vi "eHS Matrix Generation Main (Advanced).vi"(8 "Error In":errorcluster) -> (0 "error out":errorcluster)   [LabVIEW 2017]
doc: "Provides a template UI example which demonstrates how to incorporate the API in a more complex architecture (Queued Message Handler)."
uses:
  <vilib>/OPAL-RT/eHS Toolkit/eHS Matrix Generation/_Controls/eHS Core Index.ctl
  <vilib>/OPAL-RT/eHS Toolkit/eHS Matrix Generation/_Controls/eHS Form Factor.ctl
  <vilib>/OPAL-RT/eHS Toolkit/eHS Matrix Generation/_Controls/eHS Matrix Generation Session.ctl
  <vilib>/OPAL-RT/eHS Toolkit/eHS Matrix Generation/_Controls/eHS Target Information.ctl
  <vilib>/OPAL-RT/eHS Toolkit/eHS Matrix Generation/_Controls/eHS Matrix Generation Parameters.ctl
  <vilib>/OPAL-RT/eHS Toolkit/eHS Matrix Generation/_Controls/eHS Circuit Analysis Data.ctl
  <vilib>/OPAL-RT/eHS Toolkit/eHS Matrix Generation/_Controls/eHS Core Settings.ctl
  <vilib>/OPAL-RT/eHS Toolkit/eHS Matrix Generation/_Controls/eHS Model Information.ctl
  Controls/UI Data.ctl
  Controls/General UI Refs.ctl
  Controls/Info Extraction UI Refs.ctl
  Controls/Session Init UI Refs.ctl
  Controls/Matrix Gen UI Refs.ctl
  Controls/Session Reset_Close UI Refs.ctl
  Controls/Info to Add Model.ctl
  Support/ListBox/ListBox Action.ctl
  Support/Message Queue/Enqueue Message (Single).vi
  <vilib>/Utility/error.llb/Error Cluster From Error Code.vi
  <vilib>/ErrorRing/Error Ring.xnode
  Support/Message Queue/Message Queue.lvlib
  Support/User Event - Stop/User Event - Stop.lvlib
  <vilib>/OPAL-RT/eHS Toolkit/eHS Matrix Generation/eHS Matrix Generation.lvlib
panel:
  in  "TAB":T1(tab) caption="DC Source"
  in  "Add Model(s)-File":bool
  in  "eHS Listbox":i32(listbox)
  in  "Close Session":bool
  in  "Extract Model(s) Info":bool
  in  "Generate Matrix(s)":bool
  in  "Support Scenarios?":bool
  in  "Transfer Matrices":bool
  in  "Update Settings":bool
  in  "eHS Form Factor":T2=enum."eHSx64"
  in  "eHS Core Index":T3
  in  "Model Location On Disk":path
  in  "Add Model":bool
  in  "Create Session":bool
  in  "Reset Session":bool
  in  "Quit Button":bool
  in  "Target Password":string
  in  "Target Username":string="admin"
  in  "Help Button":bool
  out "?":string
  in  "Deployment Target":refnum<k21>
  in  "Get Report":bool
  out "eHS Generation Reports":string
  # "Deployment Target Settings"
  # "Model Information"
  # "Step 1: Create a session by selecting a deployment target (username and password if applicable) and click on Create Session.\nStep 2: Select *.mdl, *.slx, *.psimsch, *.cct or NI Multisim *.xml file. In addition, choose the eHS Form Factor for the generation and a Core Index for this model. \nYou can use this core index throughout the application to refer to a specific model.\nStep 3: Click on Add Model to add this model to the eHS Matrix Generation session.\nStep 4: Repeat step 2 & 3 if you want to generate more then one eHS matrix.\nStep 5: Click on Extract Model(s). This can take several minutes. The information extraction results will be displayed in the consoles to the right.\nStep 6 (Optional): Press the Update Settings button to change some of the matrix generation parameters before generating them.\nStep 7: Click on Generate Matrix(s). A eHS matrix will be generated for each model that was loaded into the session.\nStep 8: Once the matrices have been generated, you can transfer the matrices to the deplayment target by clicking on the Transfer Matrices button. \nStep 9: At this point, you can update the setting and generate a new set of matrices (Update Settings), you can reset the session (Reset Session), you can close \nthe current session (Close Session), or you can stop the application (Quit). \n \nBefore running this VI please note that:\n\n1- Before starting the real-time simulation, users need to define the circuit configuration, using an appropriate circuit editor. \nThe following circuit editors are supported by OPAL-RT TECHNOLOGIES:           \n                - Matlab/Simulink SimPowwerSystems (SPS)  (*.mdl or *.slx)\n                - Matlab/Simulink PLECS blockset  (*.mdl or *.slx)\n                - PSIM  (*.psimsch or *.cct)\n                - NI Multisim (xml output *.xml)\n\n2- PSIM and NI Multisim users have to install\t32-bit version of MATLAB® Runtime version 9.0 (R2015b) availible at:\n                                 http://www.mathworks.com/products/compiler/mcr/index.html\n\n3- Please also note that you need to have valid licence of one of the mentioned circuit editors to be able to generate the eSH matrix. In other words the users \nwho want to select SimPowerSystem (SPS) model must be have valid licence of Matlab/Simulink and SPS toolbox, the users who want to select PLECS blockset \nmodel must be have valid licence of Matlab/Simulink and PLECS blockset, the users who want to select PSIM model must be have valid licence off PSIM, and the users who want to generate and select the NI Multism xml file must be have valid licence of NI Multisim. If you don't have valid license of the \nmentioned circuit editors, you can only select prebuilt xml files."
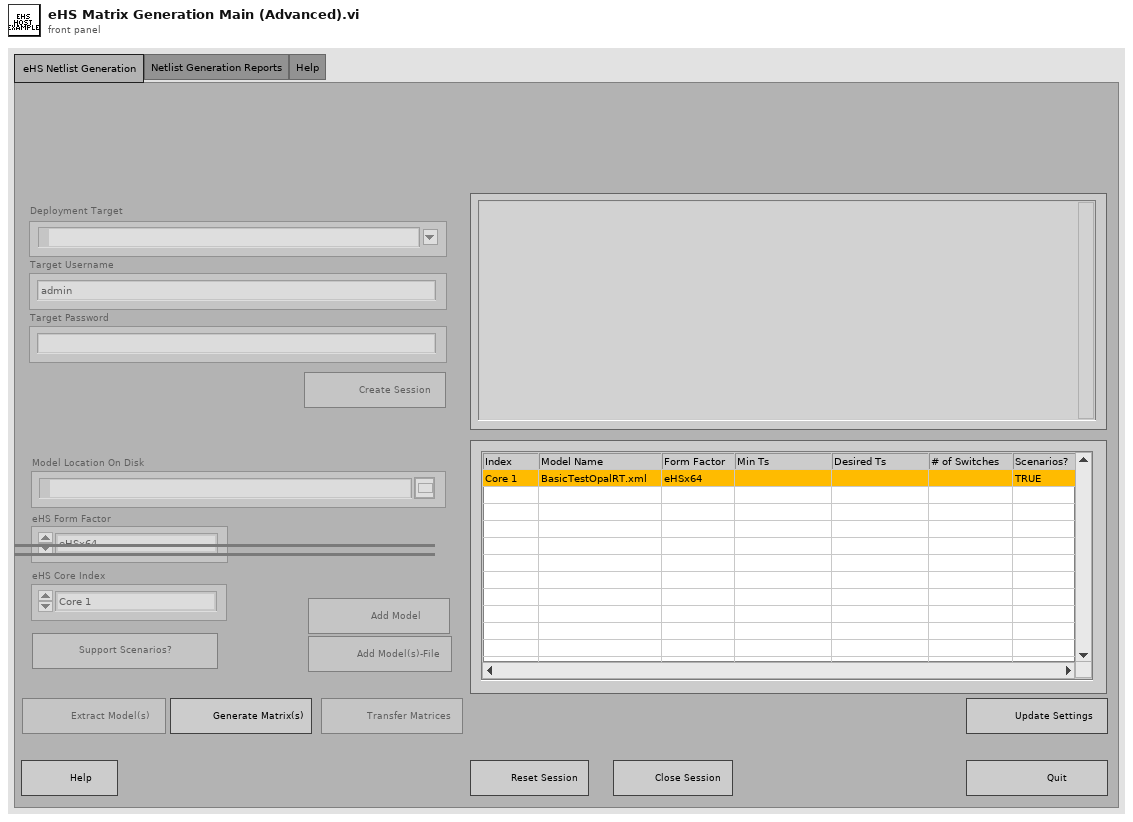
[diagram p1: front panel]
types:
  T1 = enum32{"eHS Netlist Generation ", "Netlist Generation Reports", "Help"}
  T2 = typedef "OPAL-RT eHS.lvlib/eHS Matrix Generation.lvlib/eHS Form Factor.ctl" = enum16{"eHSx16", "eHSx32", "eHSx64"}
  T3 = typedef "OPAL-RT eHS.lvlib/eHS Matrix Generation.lvlib/eHS Core Index.ctl" = enum16{"Core 1", "Core 2", "Core 3", "Core 4", "Core 5", "Core 6", "Core 7", "Core 8", "Core 9", "Core 10"}
  T4 = typedef "UI Data.ctl" = cluster{"Transfer Netlist(s)":refnum<vi>, "General Refs":T5, "Info Extraction Refs":T6, "Session Init Refs":T7, "Matrix Gen Refs":T8, "Session R\\C Refs":T9, "eHS Listbox":refnum<vi>}
  T5 = typedef "General UI Refs.ctl" = cluster{"Help":refnum<vi>, "Quit":refnum<vi>}
  T6 = typedef "Info Extraction UI Refs.ctl" = cluster{"Support Scenarios?":refnum<vi>, "Add Model":refnum<vi>, "Extract Model(s) Info":refnum<vi>, "Model Location":refnum<vi>, "Add Model(s)-File":refnum<vi>, "eHS Core Index":refnum<vi>, "eHS Form Factor":refnum<vi>}
  T7 = typedef "Session Init UI Refs.ctl" = cluster{"Create Session":refnum<vi>, "Password":refnum<vi>, "Username":refnum<vi>, "Deployment Target":refnum<vi>}
  T8 = typedef "Matrix Gen UI Refs.ctl" = cluster{"Update Settings":refnum<vi>, "Generate Matrix(s)":refnum<vi>}
  T9 = typedef "Session Reset_Close UI Refs.ctl" = cluster{"Reset Session":refnum<vi>, "Close Session":refnum<vi>}
  T10 = typedef "OPAL-RT eHS.lvlib/eHS Matrix Generation.lvlib/eHS Target Information.ctl" = cluster{"Deployment Target":refnum<k21>, "Username":string, "Password":string}
  T11 = typedef "Info to Add Model.ctl" = cluster{"eHS Core Settings":T12, "eHS Model Information":T13}
  T12 = typedef "OPAL-RT eHS.lvlib/eHS Matrix Generation.lvlib/eHS Core Settings.ctl" = cluster{"eHS Form Factor":T2, "eHS Core Index":T3}
  T13 = typedef "OPAL-RT eHS.lvlib/eHS Matrix Generation.lvlib/eHS Model Information.ctl" = cluster{"Model File Path":path, "Model Name":string, "Model File Extension":string, "Senarios?":bool}
  T14 = enum8{"Enabled", "Disabled", "Disabled and Grayed Out"}
  T15 = typedef "ListBox Action.ctl" = enum16{"Add", "Overwrite"}
  T16 = typedef "Message Queue.lvlib/All Message Queues.ctl" = cluster{"UI":refnum<queue>}
  T17 = typedef "OPAL-RT eHS.lvlib/eHS Matrix Generation.lvlib/eHS Circuit Analysis Data.ctl" = cluster{"Number of Switches":string, "Desired Ts":string, "Gs":dbl[], "Min Ts":string}
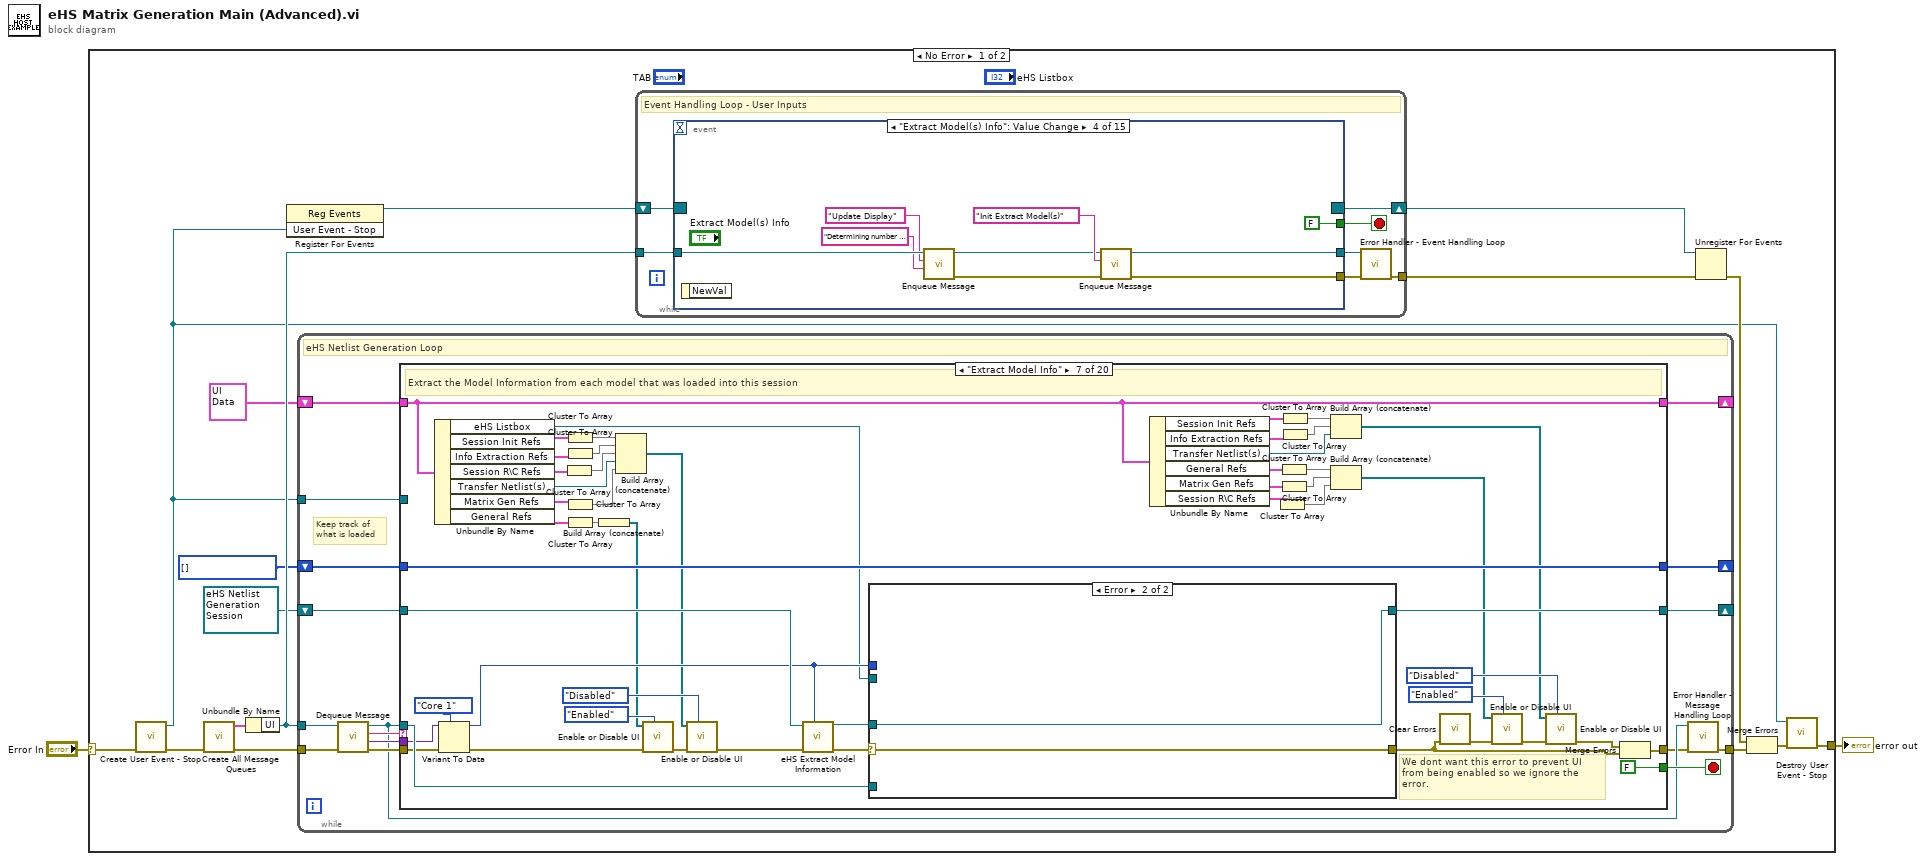
[diagram p0: block diagram]
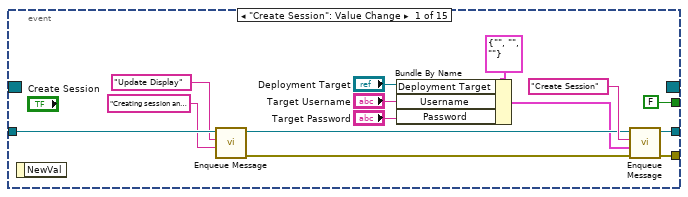
[diagram p2: hidden frame]
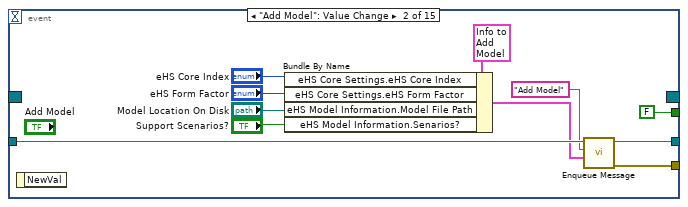
[diagram p3: hidden frame]
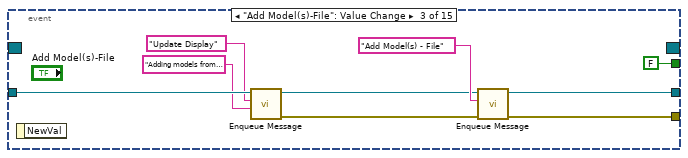
[diagram p4: hidden frame]
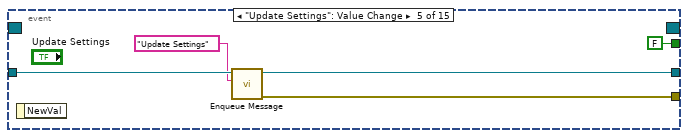
[diagram p5: hidden frame]
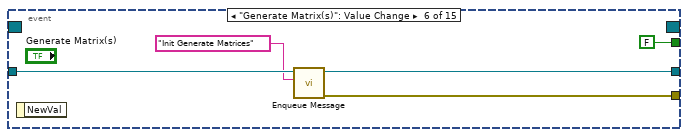
[diagram p6: hidden frame]
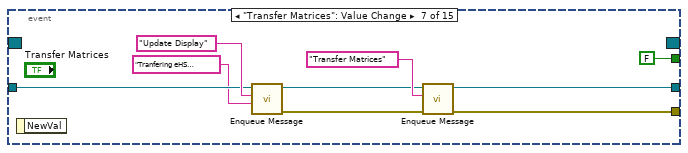
[diagram p7: hidden frame]
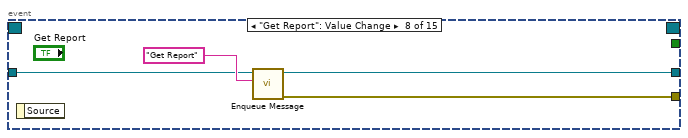
[diagram p8: hidden frame]
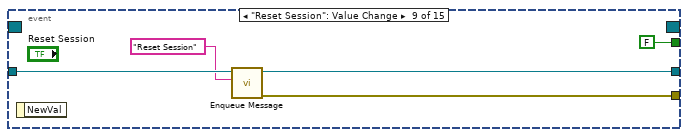
[diagram p9: hidden frame]
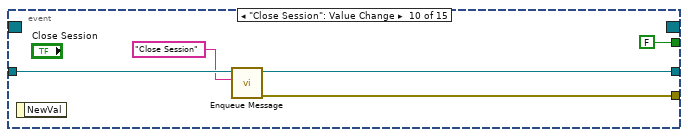
[diagram p10: hidden frame]
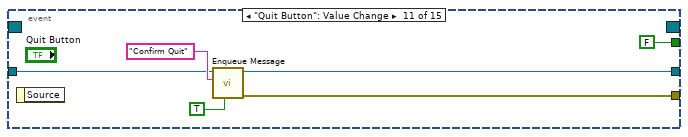
[diagram p11: hidden frame]
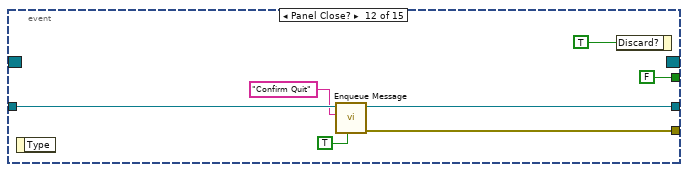
[diagram p12: hidden frame]
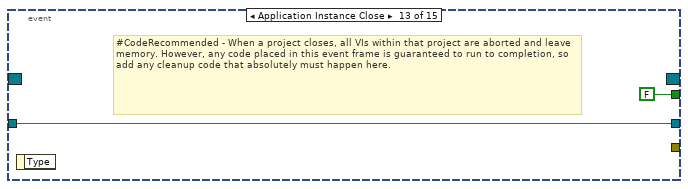
[diagram p13: hidden frame]
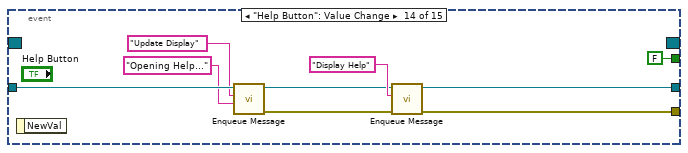
[diagram p14: hidden frame]
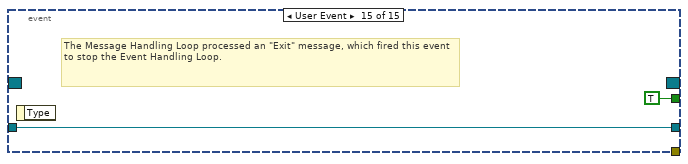
[diagram p15: hidden frame]
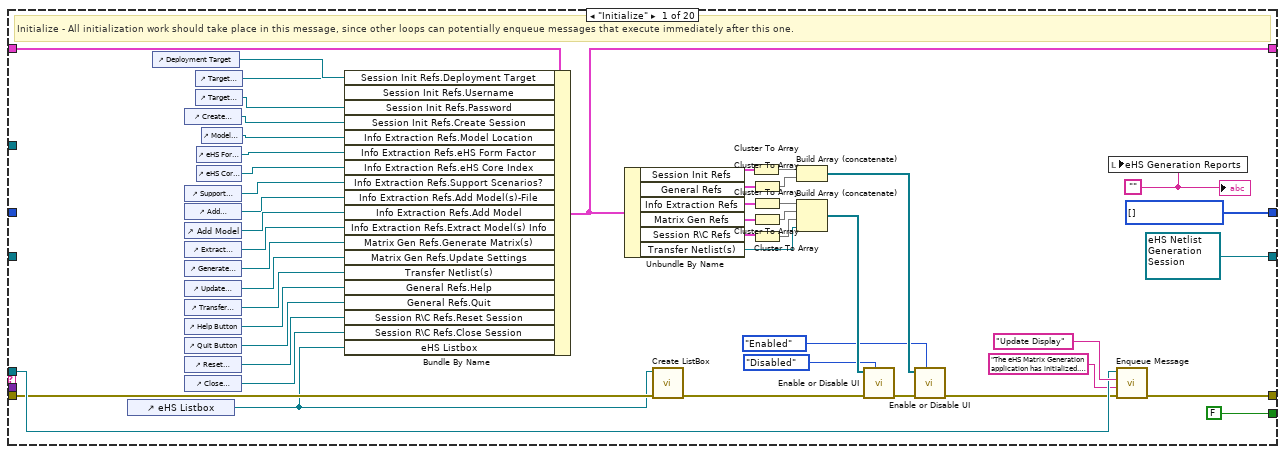
[diagram p16: hidden frame]
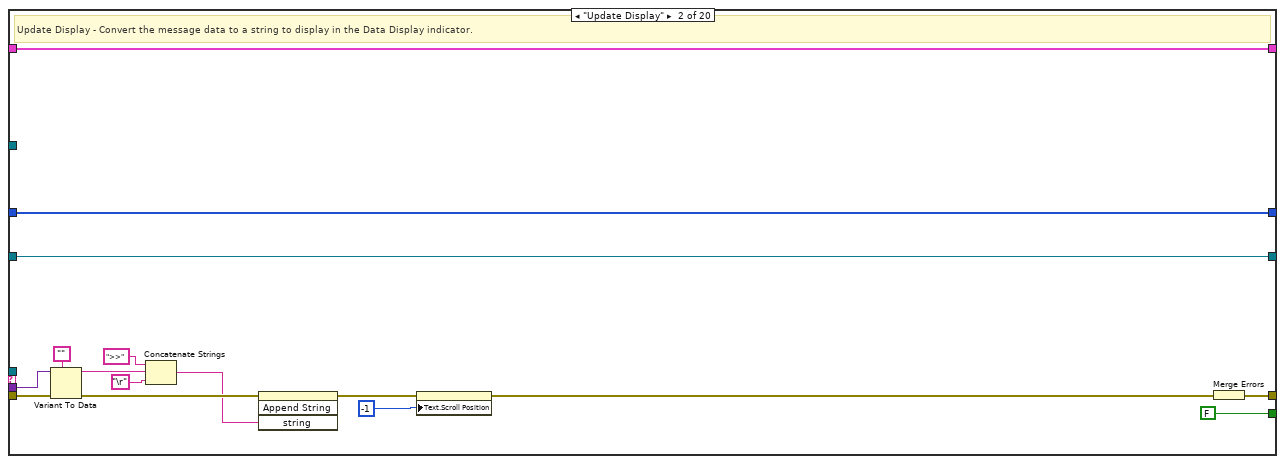
[diagram p17: hidden frame]
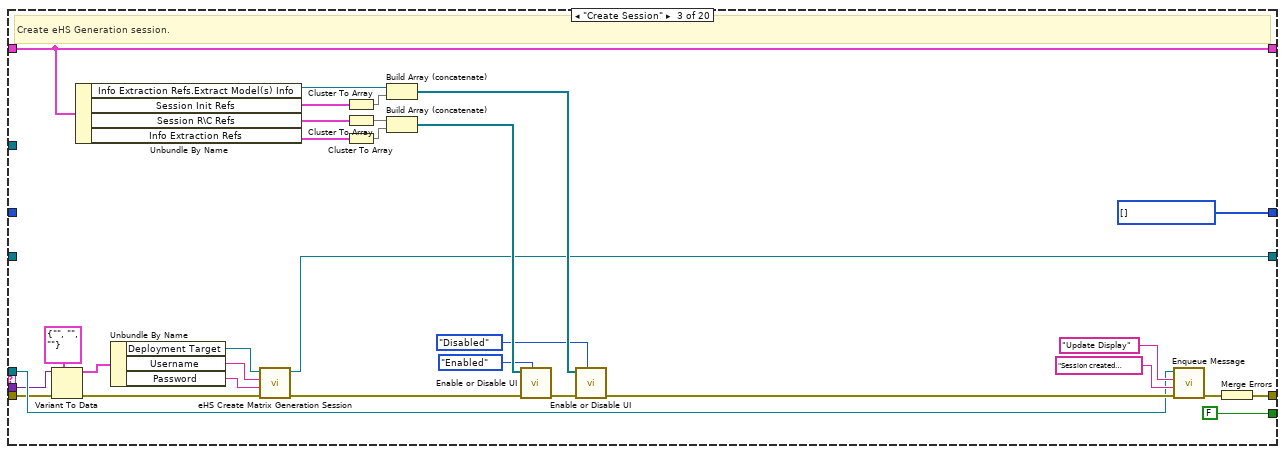
[diagram p18: hidden frame]
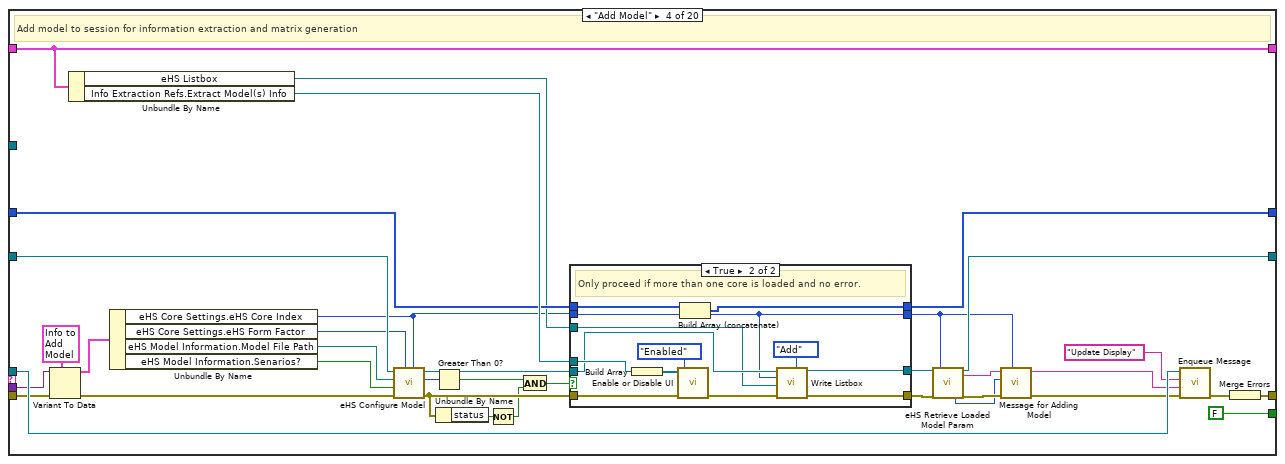
[diagram p19: hidden frame]
diagram:
  n1 = case shown="No Error" "Error In" {
    selector: "Error In" -> [w3 w781]
    tunnel: [w4 w781] -> w2
    frame No Error {
      w5 = T3[] [] items=["Core 1", "Core 2", "Core 3", "Core 4", "Core 5", "Core 6", "Core 7", "Core 8", "Core 9", "Core 10"]
      n2 = call "Create User Event - Stop.vi"("Error In"=w3) -> ("Error out"=w14:errorcluster, "User Event - Stop"=w8:refnum<user-event>)  [unwired: 9 in]
      n3 = call "Create All Message Queues.vi"("Error In"=w14) -> ("Error Out"=w18:errorcluster, "Message Queues Out"=w17:T16)  [unwired: 9 in]
      n4 = Unbundle By Name(w17) -> ("UI"=w15:refnum<queue>)
      n5 = register-events(w8) -> (reference out=w9:refnum<event-registration>)  [unwired: 2 in, 1 out]
      n6 = while {
        tunnel: w15 -> [w135]
        shift-right: [w142] -> _
        shift-left: T4 {"Transfer Netlist(s)"=refnum, "General Refs"={"Help"=refnum, "Quit"=refnum}, "Info Extraction Refs"={"Support Scenarios?"=refnum, "Add Model"=refnum, "Extract Model(s) Info"=refnum, "Model Location"=refnum, "Add Model(s)-File"=refnum, "eHS Core Index"=refnum, "eHS Form Factor"=refnum}, "Session Init Refs"={"Create Session"=refnum, "Password"=refnum, "Username"=refnum, "Deployment Target"=refnum}, "Matrix Gen Refs"={"Update Settings"=refnum, "Generate Matrix(s)"=refnum}, "Session R\\C Refs"={"Reset Session"=refnum, "Close Session"=refnum}, "eHS Listbox"=refnum} ("Data Cluster") -> [w143]
        tunnel: w8 -> [w140]
        tunnel: w18 -> [w139]
        tunnel: [w133] -> w16
        shift-right: [w130] -> _
        shift-left: refnum<data-value> refnum ("eHS Matrix Generation Session Ref") -> [w131]
        shift-right: [w128] -> _
        shift-left: w5 -> [w129]
        stop <- w141 stop-if-true
        # "Keep track of \nwhat is loaded"
        # "eHS Netlist Generation Loop"
        n7 = call "Dequeue Message.vi"("error in (no error)"=w139, "Message Queue"=w135) -> ("error out"=w138:errorcluster, "Message Data"=w136:variant, "Message"=w137:string, "dup Message Queue"=w134:refnum<queue>)  [unwired: 6 in]
        n8 = case "Message Cases" shown="\"Extract Model Info\"" w137 {
          selector: w137 -> [_ _ _ _ _ _ _ _ _ _ _ _ _ _ _ _ _ _ _ w771]
          tunnel: w134 -> [w188 _ w222 w270 w307 w342 w413 w450 w500 w547 w585 w645 w679 w699 _ w732 w753 _ _ _]
          tunnel: w138 -> [w148 w205 w215 w247 w312 w349 w412 w475 w507 w567 w617 w640 w675 w702 w719 w731 w748 w763 w767 _]
          tunnel: [w191 w206 w238 w274 w315 w363 w371 w445 w520 w575 w586 w661 w695 w700 w723 w739 w751 w757 w765 w772] -> w132
          tunnel: w143 -> [w190 w207 w228 w265 w302 w352 w389 w461 w510 w538 w595 w642 w677 w706 w724 w740 w752 w762 w766 w773]
          tunnel: [w171 w207 w228 w265 w302 w352 w389 w461 w510 w538 w595 w642 w677 w706 w724 w740 w752 w762 w766 w773] -> w142
          tunnel: [FALSE FALSE FALSE FALSE FALSE FALSE FALSE FALSE FALSE FALSE FALSE FALSE FALSE _ FALSE FALSE TRUE FALSE FALSE FALSE] -> w141
          tunnel: w136 -> [_ w204 w212 w245 _ _ w411 _ _ w566 _ _ _ _ _ _ w745 w761 _ _]
          tunnel: w140 -> [_ _ _ _ _ _ _ _ _ _ _ _ _ _ _ _ w750 _ _ _]
          tunnel: w131 -> [_ w199 _ w272 w313 w345 w416 w485 w503 w569 w612 w641 w676 w697 w720 w735 _ w755 _ w768]
          tunnel: [refnum<data-value> refnum ("eHS Matrix Generation Session Ref") w199 w220 w259 w303 w345 w415 w484 w503 w568 w611 w638 refnum<data-value> refnum ("eHS Matrix Generation Session Ref") w697 w720 w735 refnum<data-value> refnum ("eHS Matrix Generation Session Ref") w755 _ w768] -> w130
          tunnel: w129 -> [_ w198 _ w262 _ w343 w408 w453 w501 w570 w610 _ _ w696 w721 w725 _ w754 _ w769]
          tunnel: [w149 w198 w216 w263 w295 w343 w408 w453 w501 w570 w610 w636 w666 w696 w721 w725 w741 w754 _ w769] -> w128
          frame "Initialize" {
            w149 = T3[] [] items=["Core 1", "Core 2", "Core 3", "Core 4", "Core 5", "Core 6", "Core 7", "Core 8", "Core 9", "Core 10"]
            w144 = ""
            # "Initialize - All initialization work should take place in this message, since other loops can potentially enqueue messages that execute immediately after this one."
            n9 = control-ref of="eHS Listbox"() -> (w146:refnum<vi>)
            n10 = control-ref of="Deployment Target"() -> (w186:refnum<vi>)
            n11 = control-ref of="Create Session"() -> (w183:refnum<vi>)
            n12 = control-ref of="Support Scenarios?"() -> (w179:refnum<vi>)
            n13 = control-ref of="Add Model(s)-File"() -> (w145:refnum<vi>)
            n14 = control-ref of="Add Model"() -> (w178:refnum<vi>)
            n15 = control-ref of="Extract Model(s) Info"() -> (w177:refnum<vi>)
            n16 = control-ref of="Generate Matrix(s)"() -> (w176:refnum<vi>)
            n17 = control-ref of="Update Settings"() -> (w175:refnum<vi>)
            n18 = control-ref of="Transfer Matrices"() -> (w174:refnum<vi>)
            n19 = control-ref of="Help Button"() -> (w173:refnum<vi>)
            n20 = control-ref of="Quit Button"() -> (w172:refnum<vi>)
            n21 = control-ref of="Reset Session"() -> (w156:refnum<vi>)
            n22 = control-ref of="Close Session"() -> (w155:refnum<vi>)
            n23 = control-ref of="Target Username"() -> (w185:refnum<vi>)
            n24 = control-ref of="Target Password"() -> (w184:refnum<vi>)
            n25 = control-ref of="eHS Form Factor"() -> (w181:refnum<vi>)
            n26 = control-ref of="eHS Core Index"() -> (w180:refnum<vi>)
            n27 = control-ref of="Model Location On Disk"() -> (w182:refnum<vi>)
            n28 = Bundle By Name(cluster=w190, "Session Init Refs.Deployment Target"=w186, "Session Init Refs.Username"=w185, "Session Init Refs.Password"=w184, "Session Init Refs.Create Session"=w183, "Info Extraction Refs.Model Location"=w182, "Info Extraction Refs.eHS Form Factor"=w181, "Info Extraction Refs.eHS Core Index"=w180, "Info Extraction Refs.Support Scenarios?"=w179, "Info Extraction Refs.Add Model(s)-File"=w145, "Info Extraction Refs.Add Model"=w178, "Info Extraction Refs.Extract Model(s) Info"=w177, "Matrix Gen Refs.Generate Matrix(s)"=w176, "Matrix Gen Refs.Update Settings"=w175, "Transfer Netlist(s)"=w174, "General Refs.Help"=w173, "General Refs.Quit"=w172, "Session R\\C Refs.Reset Session"=w156, "Session R\\C Refs.Close Session"=w155, "eHS Listbox"=w146) -> (w171:T4)
            n29 = Unbundle By Name(w171) -> ("Session Init Refs"=w169:T7, "General Refs"=w170:T5, "Info Extraction Refs"=w168:T6, "Matrix Gen Refs"=w153:T8, "Session R\\C Refs"=w152:T9, "Transfer Netlist(s)"=w154:refnum<vi>)
            n30 = call "Create ListBox.vi"("Error In"=w148, "Multicolumn Listbox Ref In"=w146) -> ("Error Out"=w147:errorcluster)  [unwired: 8 in, 1 out]
            n31 = Cluster To Array(cluster=w169) -> (array=w167:refnum<vi>[])
            n32 = Cluster To Array(cluster=w170) -> (array=w166:refnum<vi>[])
            n33 = Cluster To Array(cluster=w168) -> (array=w164:refnum<vi>[])
            n34 = Cluster To Array(cluster=w153) -> (array=w165:refnum<vi>[])
            n35 = Cluster To Array(cluster=w152) -> (array=w151:refnum<vi>[])
            n36 = Build Array (concatenate)(w167, w166) -> (w159:refnum<vi>[])
            n37 = Build Array (concatenate)(w164, w165, w151, w154) -> (w163:refnum<vi>[])
            n38 = call "Enable or Disable UI.vi"("Action"=T14."Disabled", "Error In"=w147, "Control Refs"=w163) -> ("Error Out"=w161:errorcluster)  [unwired: 8 in]
            n39 = call "Enable or Disable UI.vi"("Action"=T14."Enabled", "Error In"=w161, "Control Refs"=w159) -> ("Error Out"=w160:errorcluster)  [unwired: 8 in]
            n40 = local write "eHS Generation Reports"(w144) -> ()
            n41 = call-poly "Enqueue Message.vi"("Error In"=w160, "Message Data"="The eHS Matrix Generation application has initialized. Please create a new session." ("Initial Message"), "Message"="Update Display", "Message Queue"=w188) -> ("Error Out"=w191:errorcluster)  [unwired: 6 in, 1 out]
            "?" <- w144
          }
          frame "Update Display" {
            # "Update Display - Convert the message data to a string to display in the Data Display indicator."
            n42 = Variant To Data(error in=w205, type="", Variant=w204) -> (data=w202:string, error out=w196:errorcluster)
            n43 = Concatenate Strings(">>" ("string"), w202, "\r") -> (w195:string)
            n44 = invoke class="Str" method="Append String"(error in=w196, "string"=w195) -> (error out=w194:errorcluster)  [unwired: 2 in, 3 out]
            n45 = property class="Str"(error in=w194, "Text.Scroll Position"=-1) -> (error out=w193:errorcluster)  [unwired: 1 in, 1 out]
            n46 = Merge Errors(w193) -> (w206:errorcluster)
          }
          frame "Create Session" {
            w216 = T3[] [] items=["Core 1", "Core 2", "Core 3", "Core 4", "Core 5", "Core 6", "Core 7", "Core 8", "Core 9", "Core 10"]
            # "Create eHS Generation session."
            n47 = Variant To Data(error in=w215, type=T10 {"Deployment Target"="", "Username"="", "Password"=""} ("eHS Target Information"), Variant=w212) -> (data=w211:T10, error out=w214:errorcluster)
            n48 = Unbundle By Name(w228) -> ("Info Extraction Refs.Extract Model(s) Info"=w217:refnum<vi>, "Session Init Refs"=w234:T7, "Session R\\C Refs"=w226:T9, "Info Extraction Refs"=w219:T6)
            n49 = Unbundle By Name(w211) -> ("Deployment Target"=w210:refnum<k21>, "Username"=w209:string, "Password"=w208:string)
            n50 = call <vilib>:"eHS Create Matrix Generation Session.vi"("Error In"=w214, "Target Password"=w208, "Target Username"=w209, "Deployment Target"=w210) -> ("Error Out"=w221:errorcluster, "eHS Matrix Generation Session Ref"=w220:refnum<data-value>)  [unwired: 6 in]
            n51 = Cluster To Array(cluster=w234) -> (array=w233:refnum<vi>[])
            n52 = Cluster To Array(cluster=w226) -> (array=w225:refnum<vi>[])
            n53 = Cluster To Array(cluster=w219) -> (array=w218:refnum<vi>[])
            n54 = Build Array (concatenate)(w217, w233) -> (w230:refnum<vi>[])
            n55 = Build Array (concatenate)(w225, w218) -> (w232:refnum<vi>[])
            n56 = call "Enable or Disable UI.vi"("Action"=T14."Enabled", "Error In"=w221, "Control Refs"=w232) -> ("Error Out"=w227:errorcluster)  [unwired: 8 in]
            n57 = call "Enable or Disable UI.vi"("Action"=T14."Disabled", "Error In"=w227, "Control Refs"=w230) -> ("Error Out"=w223:errorcluster)  [unwired: 8 in]
            n58 = call-poly "Enqueue Message.vi"("Error In"=w223, "Message Data"="Session created successfully. Ready to add models for matrix generation." ("Message"), "Message"="Update Display", "Message Queue"=w222) -> ("Error Out"=w224:errorcluster)  [unwired: 6 in, 1 out]
            n59 = Merge Errors(w224) -> (w238:errorcluster)
          }
          frame "Add Model" {
            # "Add model to session for information extraction and matrix generation"
            n60 = Variant To Data(error in=w247, type=T11 {"eHS Core Settings"={"eHS Form Factor"=enum."eHSx16", "eHS Core Index"=enum."Core 1"}, "eHS Model Information"={"Model File Path"=path "", "Model Name"="", "Model File Extension"="", "Senarios?"=FALSE}} ("Info to Add Model"), Variant=w245) -> (data=w243:T11, error out=w246:errorcluster)
            n61 = Unbundle By Name(w265) -> ("eHS Listbox"=w248:refnum<vi>, "Info Extraction Refs.Extract Model(s) Info"=w264:refnum<vi>)
            n62 = Unbundle By Name(w243) -> ("eHS Core Settings.eHS Core Index"=w242:T3, "eHS Core Settings.eHS Form Factor"=w241:T2, "eHS Model Information.Model File Path"=w240:path, "eHS Model Information.Senarios?"=w239:bool)
            n63 = call <vilib>:"eHS Configure Model.vi"("eHS Core Index"=w242, "eHS Form Factor"=w241, "Error In"=w246, "Support Senarios?"=w239, "Model File Path"=w240, "eHS Matrix Generation Session Ref In"=w272) -> ("Error Out"=w253:errorcluster, "Number of Cores Loaded"=w266:i32, "eHS Matrix Generation Session Ref Out"=w249:refnum<data-value>)  [unwired: 3 in]
            n64 = Greater Than 0?(x=w266) -> (x > 0?=w255:bool)
            n65 = Unbundle By Name(w253) -> ("status"=w252:bool)
            n66 = Not(x=w252) -> (.not. x?=w251:bool)
            n67 = And(x=w255, y=w251) -> (x .and. y?=w254:bool)
            n68 = case shown="True" w254 {
              tunnel: w242 -> [w276 w281]
              tunnel: w262 -> [w278 w291]
              tunnel: [w278 w290] -> w263
              tunnel: w253 -> [w277 w288]
              tunnel: [w277 w284] -> w261
              tunnel: w264 -> [_ w286]
              tunnel: [w276 w281] -> w256
              tunnel: [w275 w283] -> w250
              tunnel: w249 -> [w275 w282]
              tunnel: w248 -> [_ w280]
              frame False {
                # "Do nothing if no cores are loaded or error"
              }
              frame True {
                # "Only proceed if more than one core is loaded and no error."
                n69 = Build Array(w286) -> (w289:refnum<vi>[])
                n70 = call "Enable or Disable UI.vi"("Action"=T14."Enabled", "Error In"=w288, "Control Refs"=w289) -> ("Error Out"=w285:errorcluster)  [unwired: 8 in]
                n71 = Build Array (concatenate)(w291, w281) -> (w290:T3[])
                n72 = call "Write Listbox.vi"("Action"=ListBox_Action."Add" ("ListBox Action"), "eHS Core Index"=w281, "Error In"=w285, "Multicolumn Listbox Ref In"=w280, "eHS Matrix Generation Session Ref In"=w282) -> ("Error Out"=w284:errorcluster, "eHS Matrix Generation Session Ref Out"=w283:refnum<data-value>)  [unwired: 4 in, 1 out]
              }
            }
            n73 = call <vilib>:"eHS Retrieve Loaded Model Param.vi"("eHS Matrix Generation Session Ref In"=w250, "Error In"=w261, "eHS Core Index"=w256) -> ("Number of Loaded Models"=w257:i32, "eHS Matrix Generation Session Ref Out"=w259:refnum<data-value>, "Model Name"=w258:string, "Error Out"=w260:errorcluster)  [unwired: 10 in, 3 out]
            n74 = call "Message for Adding Model.vi"("eHS Core Index"=w256, "Error In"=w260, "Number of Loaded Models"=w257, "Model File Name"=w258) -> ("Error Out"=w267:errorcluster, "Message"=w268:string)  [unwired: 6 in]
            n75 = call-poly "Enqueue Message.vi"("Error In"=w267, "Message Data"=w268, "Message"="Update Display", "Message Queue"=w270) -> ("Error Out"=w271:errorcluster)  [unwired: 6 in, 1 out]
            n76 = Merge Errors(w271) -> (w274:errorcluster)
          }
          frame "Add Model(s) - File" {
            # "Duplicate this frame when creating new messages.  Change this comment in the duplicated frame to describe this message."
            n77 = Unbundle By Name(w302) -> ("Info Extraction Refs.Extract Model(s) Info"=w301:refnum<vi>, "eHS Listbox"=w293:refnum<vi>)
            n78 = call "Get Model(s) Config File.vi"("Error In"=w312, "eHS Matrix Generation Session Ref In"=w313) -> ("Error Out"=w310:errorcluster, "Model(s) Config File Path"=w309:path, "eHS Matrix Generation Session Ref Out"=w311:refnum<data-value>)  [unwired: 7 in]
            n79 = call <vilib>:"eHS Configure Model(s) from File.vi"("Error In"=w310, "Model Config File Path"=w309, "eHS Matrix Generation Session Ref In"=w311) -> ("Error Out"=w292:errorcluster, "Loaded Core Indexes"=w295:T3[], "eHS Matrix Generation Session Ref Out"=w294:refnum<data-value>, "Number of Cores Loaded"=w304:i32)  [unwired: 5 in]
            n80 = Greater Than 0?(x=w304) -> (x > 0?=w298:bool)
            n81 = Build Array(w301) -> (w300:refnum<vi>[])
            n82 = for {
              shift-right: [w318] -> w297
              shift-left: w292 -> [w316]
              shift-right: [w322] -> w296
              shift-left: w294 -> [w323]
              tunnel: w295 -> [w321] mode=indexing
              tunnel: w293 -> [w320]
              n83 = call "Write Listbox.vi"("Action"=ListBox_Action."Add" ("ListBox Action"), "eHS Core Index"=w321, "Multicolumn Listbox Ref In"=w320, "eHS Matrix Generation Session Ref In"=w323) -> ("Error Out"=w317:errorcluster, "eHS Matrix Generation Session Ref Out"=w322:refnum<data-value>)  [unwired: 5 in, 1 out]
              n84 = Merge Errors(w316, w317) -> (w318:errorcluster)
            }
            n85 = case shown="True" w298 {
              tunnel: [w325 w328] -> w305
              tunnel: w296 -> [w324 w331]
              tunnel: w297 -> [w325 w326]
              tunnel: [w324 w331] -> w303
              tunnel: w300 -> [_ w329]
              frame False {
              }
              frame True {
                n86 = call "Enable or Disable UI.vi"("Action"=T14."Enabled", "Control Refs"=w329) -> ("Error Out"=w327:errorcluster)  [unwired: 9 in]
                n87 = Merge Errors(w326, w327) -> (w328:errorcluster)
              }
            }
            n88 = call-poly "Enqueue Message.vi"("Error In"=w305, "Message Data"="Models successfully added to the session." ("Message"), "Message"="Update Display", "Message Queue"=w307) -> ("Error Out"=w306:errorcluster)  [unwired: 6 in, 1 out]
            n89 = Merge Errors(w306) -> (w315:errorcluster)
          }
          frame "Init Extract Model(s)" {
            # "Detemine how many models must be operated on for the information extraction process."
            n90 = Unbundle By Name(w352) -> ("Session Init Refs"=w361:T7, "Info Extraction Refs"=w360:T6, "Session R\\C Refs"=w357:T9, "Transfer Netlist(s)"=w355:refnum<vi>, "General Refs"=w354:T5)
            n91 = Cluster To Array(cluster=w357) -> (array=w356:refnum<vi>[])
            n92 = Cluster To Array(cluster=w361) -> (array=w359:refnum<vi>[])
            n93 = Cluster To Array(cluster=w360) -> (array=w358:refnum<vi>[])
            n94 = Cluster To Array(cluster=w354) -> (array=w353:refnum<vi>[])
            n95 = Build Array (concatenate)(w353) -> (w347:refnum<vi>[])
            n96 = Build Array (concatenate)(w359, w358, w356, w355) -> (w346:refnum<vi>[])
            n97 = call "Enable or Disable UI.vi"("Action"=T14."Enabled", "Error In"=w349, "Control Refs"=w347) -> ("Error Out"=w348:errorcluster)  [unwired: 8 in]
            n98 = call "Enable or Disable UI.vi"("Action"=T14."Disabled", "Error In"=w348, "Control Refs"=w346) -> ("Error Out"=w344:errorcluster)  [unwired: 8 in]
            n99 = for {
              tunnel: w343 -> [w367] mode=indexing
              tunnel: w342 -> [w368]
              shift-right: [w365] -> w341
              shift-left: w344 -> [w369]
              tunnel: [w364] -> w340
              n100 = call-poly "Enqueue Message.vi"("Error In"=w369, "Message Data"=w367, "Message"="Extract Model Info", "Message Queue"=w368) -> ("Error Out"=w365:errorcluster, "dup Message Queue"=w364:refnum<queue>)  [unwired: 6 in]
            }
            n101 = call-poly "Enqueue Message.vi"("Priority Message? (F)"=TRUE, "Error In"=w341, "Message Data"="Extraction starting. This can take several minutes..." ("Message"), "Message"="Update Display", "Message Queue"=w340) -> ("Error Out"=w336:errorcluster, "dup Message Queue"=w335:refnum<queue>)  [unwired: 5 in]
            n102 = call-poly "Enqueue Message.vi"("Error In"=w336, "Message Data"="Extraction finished." ("Message"), "Message"="Update Display", "Message Queue"=w335) -> ("Error Out"=w334:errorcluster)  [unwired: 6 in, 1 out]
            n103 = Merge Errors(w334) -> (w363:errorcluster)
          }
          frame "Extract Model Info" {
            # "We dont want this error to prevent UI from being enabled so we ignore the error."
            # "Extract the Model Information from each model that was loaded into this session"
            n104 = Unbundle By Name(w389) -> ("eHS Listbox"=w374:refnum<vi>, "Session Init Refs"=w407:T7, "Info Extraction Refs"=w406:T6, "Session R\\C Refs"=w403:T9, "Transfer Netlist(s)"=w401:refnum<vi>, "Matrix Gen Refs"=w376:T8, "General Refs"=w377:T5)
            n105 = Variant To Data(error in=w412, type=eHS_Core_Index."Core 1" ("eHS Core Index"), Variant=w411) -> (data=w409:T3, error out=w383:errorcluster)
            n106 = Cluster To Array(cluster=w403) -> (array=w402:refnum<vi>[])
            n107 = Cluster To Array(cluster=w407) -> (array=w405:refnum<vi>[])
            n108 = Cluster To Array(cluster=w406) -> (array=w404:refnum<vi>[])
            n109 = Cluster To Array(cluster=w376) -> (array=w375:refnum<vi>[])
            n110 = Cluster To Array(cluster=w377) -> (array=w400:refnum<vi>[])
            n111 = Build Array (concatenate)(w400) -> (w398:refnum<vi>[])
            n112 = Build Array (concatenate)(w405, w404, w402, w401, w375) -> (w399:refnum<vi>[])
            n113 = call "Enable or Disable UI.vi"("Action"=T14."Enabled", "Error In"=w383, "Control Refs"=w398) -> ("Error Out"=w417:errorcluster)  [unwired: 8 in]
            n114 = call "Enable or Disable UI.vi"("Action"=T14."Disabled", "Error In"=w417, "Control Refs"=w399) -> ("Error Out"=w382:errorcluster)  [unwired: 8 in]
            n115 = call <vilib>:"eHS Extract Model Information.vi"("eHS Core Index"=w409, "Error In"=w382, "eHS Matrix Generation Session Ref In"=w416) -> ("Error Out"=w381:errorcluster, "eHS Matrix Generation Session Ref Out"=w414:refnum<data-value>)  [unwired: 5 in, 2 out]
            n116 = case shown="Error" w381 {
              selector: w381 -> [w438 w441]
              tunnel: [w426 w441] -> w370
              tunnel: w414 -> [w437 w440]
              tunnel: [w424 w440] -> w415
              tunnel: w413 -> [w439 _]
              tunnel: w409 -> [w422 _]
              tunnel: w374 -> [w423 _]
              frame No Error {
                n117 = call <vilib>:"eHS Retrieve Loaded Model Param.vi"("eHS Matrix Generation Session Ref In"=w437, "Error In"=w438, "eHS Core Index"=w422) -> ("eHS Matrix Generation Session Ref Out"=w425:refnum<data-value>, "Model Name"=w433:string, "eHS Circuit Analysis Data"=w432:T17, "Error Out"=w435:errorcluster)  [unwired: 10 in, 3 out]
                n118 = Unbundle By Name(w432) -> ("Min Ts"=w430:string, "Number of Switches"=w431:string)
                n119 = call "Message for Extracting Info.vi"("eHS Core Index"=w422, "Model Name"=w433, "Minimum Ts"=w430, "Number of Switchs"=w431, "Error In"=w435) -> ("Message"=w429:string, "Error Out"=w434:errorcluster)  [unwired: 9 in]
                n120 = call-poly "Enqueue Message.vi"("Priority Message? (F)"=TRUE, "Error In"=w434, "Message Data"=w429, "Message"="Update Display", "Message Queue"=w439) -> ("Error Out"=w427:errorcluster)  [unwired: 5 in, 1 out]
                n121 = call "Write Listbox.vi"("Action"=ListBox_Action."Overwrite" ("ListBox Action"), "eHS Core Index"=w422, "Error In"=w427, "Multicolumn Listbox Ref In"=w423, "eHS Matrix Generation Session Ref In"=w425) -> ("Error Out"=w426:errorcluster, "eHS Matrix Generation Session Ref Out"=w424:refnum<data-value>)  [unwired: 4 in, 1 out]
              }
              frame Error {
              }
            }
            n122 = Unbundle By Name(w389) -> ("Session Init Refs"=w390:T7, "Info Extraction Refs"=w391:T6, "Transfer Netlist(s)"=w388:refnum<vi>, "General Refs"=w393:T5, "Matrix Gen Refs"=w380:T8, "Session R\\C Refs"=w379:T9)
            n123 = Cluster To Array(cluster=w379) -> (array=w378:refnum<vi>[])
            n124 = Cluster To Array(cluster=w393) -> (array=w394:refnum<vi>[])
            n125 = Cluster To Array(cluster=w380) -> (array=w385:refnum<vi>[])
            n126 = Cluster To Array(cluster=w390) -> (array=w386:refnum<vi>[])
            n127 = Cluster To Array(cluster=w391) -> (array=w392:refnum<vi>[])
            n128 = Build Array (concatenate)(w386, w392, w388) -> (w387:refnum<vi>[])
            n129 = Build Array (concatenate)(w394, w385, w378) -> (w384:refnum<vi>[])
            n130 = call <vilib>:"Clear Errors.vi"("error in (no error)"=w370) -> ("error out"=w373:errorcluster)  [unwired: 5 in, 1 out]
            n131 = call "Enable or Disable UI.vi"("Action"=T14."Enabled", "Error In"=w373, "Control Refs"=w384) -> ("Error Out"=w396:errorcluster)  [unwired: 8 in]
            n132 = call "Enable or Disable UI.vi"("Action"=T14."Disabled", "Error In"=w396, "Control Refs"=w387) -> ("Error Out"=w372:errorcluster)  [unwired: 8 in]
            n133 = Merge Errors(w372, w370) -> (w371:errorcluster)
          }
          frame "Update Settings" {
            # "*****Do not leave the front panel\nof this VI open when running the \nmain application"
            # "We dont want this error to prevent UI from being enabled so we ignore the error."
            # "Update the setting of each loaded model."
            n134 = Unbundle By Name(w461) -> ("eHS Listbox"=w447:refnum<vi>, "Session Init Refs"=w483:T7, "Info Extraction Refs"=w482:T6, "Session R\\C Refs"=w479:T9, "Transfer Netlist(s)"=w477:refnum<vi>, "Matrix Gen Refs"=w460:T8, "General Refs"=w458:T5)
            n135 = Cluster To Array(cluster=w483) -> (array=w481:refnum<vi>[])
            n136 = Cluster To Array(cluster=w482) -> (array=w480:refnum<vi>[])
            n137 = Cluster To Array(cluster=w479) -> (array=w478:refnum<vi>[])
            n138 = Cluster To Array(cluster=w460) -> (array=w459:refnum<vi>[])
            n139 = Cluster To Array(cluster=w458) -> (array=w457:refnum<vi>[])
            n140 = Build Array (concatenate)(w481, w480, w478, w477, w459, w457) -> (w473:refnum<vi>[])
            n141 = call "Enable or Disable UI.vi"("Action"=T14."Disabled", "Error In"=w475, "Control Refs"=w473) -> ("Error Out"=w474:errorcluster)  [unwired: 8 in]
            n142 = call "Update Settings.vi"("Multicolumn Listbox Ref In"=w447, "Error In"=w474, "eHS Matrix Generation Session Ref In"=w485) -> ("Error Out"=w442:errorcluster, "eHS Matrix Generation Session Ref Out"=w484:refnum<data-value>)  [unwired: 7 in]
            n143 = Unbundle By Name(w461) -> ("Session Init Refs"=w468:T7, "Info Extraction Refs"=w469:T6, "Transfer Netlist(s)"=w467:refnum<vi>, "General Refs"=w471:T5, "Matrix Gen Refs"=w464:T8, "Session R\\C Refs"=w463:T9)
            n144 = Cluster To Array(cluster=w463) -> (array=w462:refnum<vi>[])
            n145 = Cluster To Array(cluster=w471) -> (array=w472:refnum<vi>[])
            n146 = Cluster To Array(cluster=w464) -> (array=w465:refnum<vi>[])
            n147 = Cluster To Array(cluster=w468) -> (array=w466:refnum<vi>[])
            n148 = Cluster To Array(cluster=w469) -> (array=w470:refnum<vi>[])
            n149 = Build Array (concatenate)(w466, w470, w467) -> (w451:refnum<vi>[])
            n150 = Build Array (concatenate)(w472, w465, w462) -> (w452:refnum<vi>[])
            n151 = call <vilib>:"Clear Errors.vi"("error in (no error)"=w442) -> ("error out"=w446:errorcluster)  [unwired: 5 in, 1 out]
            n152 = call "Enable or Disable UI.vi"("Action"=T14."Enabled", "Error In"=w446, "Control Refs"=w452) -> ("Error Out"=w455:errorcluster)  [unwired: 8 in]
            n153 = call "Enable or Disable UI.vi"("Action"=T14."Disabled", "Error In"=w455, "Control Refs"=w451) -> ("Error Out"=w443:errorcluster)  [unwired: 8 in]
            n154 = Merge Errors(w443, w442) -> (w444:errorcluster)
            n155 = call-poly "Enqueue Message.vi"("Error In"=w444, "Message Data"="Update complete." ("Message"), "Message"="Update Display", "Message Queue"=w450) -> ("Error Out"=w445:errorcluster)  [unwired: 6 in, 1 out]
          }
          frame "Init Generate Matrices" {
            # "Detemine how many models must be operated on for the eHS matrix generation process."
            n156 = Unbundle By Name(w510) -> ("Session Init Refs"=w518:T7, "Info Extraction Refs"=w517:T6, "Session R\\C Refs"=w514:T9, "Transfer Netlist(s)"=w512:refnum<vi>, "Matrix Gen Refs"=w488:T8, "General Refs"=w489:T5)
            n157 = Cluster To Array(cluster=w514) -> (array=w513:refnum<vi>[])
            n158 = Cluster To Array(cluster=w518) -> (array=w516:refnum<vi>[])
            n159 = Cluster To Array(cluster=w517) -> (array=w515:refnum<vi>[])
            n160 = Cluster To Array(cluster=w488) -> (array=w487:refnum<vi>[])
            n161 = Cluster To Array(cluster=w489) -> (array=w511:refnum<vi>[])
            n162 = Build Array (concatenate)(w511) -> (w505:refnum<vi>[])
            n163 = Build Array (concatenate)(w516, w515, w513, w512, w487) -> (w504:refnum<vi>[])
            n164 = call "Enable or Disable UI.vi"("Action"=T14."Enabled", "Error In"=w507, "Control Refs"=w505) -> ("Error Out"=w506:errorcluster)  [unwired: 8 in]
            n165 = call "Enable or Disable UI.vi"("Action"=T14."Disabled", "Error In"=w506, "Control Refs"=w504) -> ("Error Out"=w502:errorcluster)  [unwired: 8 in]
            n166 = for {
              tunnel: w501 -> [w524] mode=indexing
              tunnel: w500 -> [w525]
              shift-right: [w522] -> w499
              shift-left: w502 -> [w526]
              tunnel: [w521] -> w498
              n167 = call-poly "Enqueue Message.vi"("Error In"=w526, "Message Data"=w524, "Message"="Generate eHS Matrix", "Message Queue"=w525) -> ("Error Out"=w522:errorcluster, "dup Message Queue"=w521:refnum<queue>)  [unwired: 6 in]
            }
            n168 = call-poly "Enqueue Message.vi"("Priority Message? (F)"=TRUE, "Error In"=w499, "Message Data"="Matrix generation starting. This can take several minutes..." ("Message"), "Message"="Update Display", "Message Queue"=w498) -> ("Error Out"=w494:errorcluster, "dup Message Queue"=w493:refnum<queue>)  [unwired: 5 in]
            n169 = call-poly "Enqueue Message.vi"("Error In"=w494, "Message Data"="eHS matrix generation finished." ("Message"), "Message"="Update Display", "Message Queue"=w493) -> ("Error Out"=w492:errorcluster)  [unwired: 6 in, 1 out]
            n170 = Merge Errors(w492) -> (w520:errorcluster)
          }
          frame "Generate eHS Matrix" {
            # "We dont want this error to prevent UI from being enabled so we ignore the error."
            # "Detemine how many models must be operated on for the eHS matrix generation process."
            n171 = Variant To Data(error in=w567, type=eHS_Core_Index."Core 1" ("eHS Core Index"), Variant=w566) -> (data=w548:T3, error out=w551:errorcluster)
            n172 = Unbundle By Name(w538) -> ("Session Init Refs"=w564:T7, "Info Extraction Refs"=w563:T6, "Session R\\C Refs"=w560:T9, "Transfer Netlist(s)"=w558:refnum<vi>, "Matrix Gen Refs"=w555:T8, "General Refs"=w556:T5)
            n173 = Cluster To Array(cluster=w560) -> (array=w559:refnum<vi>[])
            n174 = Cluster To Array(cluster=w564) -> (array=w562:refnum<vi>[])
            n175 = Cluster To Array(cluster=w563) -> (array=w561:refnum<vi>[])
            n176 = Cluster To Array(cluster=w555) -> (array=w554:refnum<vi>[])
            n177 = Cluster To Array(cluster=w556) -> (array=w557:refnum<vi>[])
            n178 = Build Array (concatenate)(w557) -> (w552:refnum<vi>[])
            n179 = Build Array (concatenate)(w562, w561, w559, w558, w554) -> (w553:refnum<vi>[])
            n180 = call "Enable or Disable UI.vi"("Action"=T14."Enabled", "Error In"=w551, "Control Refs"=w552) -> ("Error Out"=w571:errorcluster)  [unwired: 8 in]
            n181 = call "Enable or Disable UI.vi"("Action"=T14."Disabled", "Error In"=w571, "Control Refs"=w553) -> ("Error Out"=w550:errorcluster)  [unwired: 8 in]
            n182 = call <vilib>:"eHS Generate Matrix.vi"("eHS Core Index"=w548, "Error In"=w550, "eHS Matrix Generation Session Ref In"=w569) -> ("Error Out"=w549:errorcluster, "eHS Matrix Generation Session Ref Out"=w568:refnum<data-value>)  [unwired: 7 in]
            n183 = case shown="No Error" w549 {
              selector: w549 -> [w583 w584]
              tunnel: w548 -> [w582 _]
              tunnel: w547 -> [w580 _]
              tunnel: [w577 w584] -> w527
              frame No Error {
                n184 = call "Message for Generation.vi"("Error In"=w583, "eHS Core Index"=w582) -> ("Error Out"=w581:errorcluster, "Message"=w579:string)  [unwired: 8 in]
                n185 = call-poly "Enqueue Message.vi"("Priority Message? (F)"=TRUE, "Error In"=w581, "Message Data"=w579, "Message"="Update Display", "Message Queue"=w580) -> ("Error Out"=w577:errorcluster)  [unwired: 5 in, 1 out]
              }
              frame Error {
              }
            }
            n186 = Unbundle By Name(w538) -> ("Session Init Refs"=w546:T7, "Info Extraction Refs"=w545:T6, "Matrix Gen Refs"=w537:T8, "General Refs"=w542:T5, "Session R\\C Refs"=w536:T9, "Transfer Netlist(s)"=w530:refnum<vi>)
            n187 = Cluster To Array(cluster=w546) -> (array=w544:refnum<vi>[])
            n188 = Cluster To Array(cluster=w545) -> (array=w543:refnum<vi>[])
            n189 = Cluster To Array(cluster=w537) -> (array=w535:refnum<vi>[])
            n190 = Cluster To Array(cluster=w542) -> (array=w534:refnum<vi>[])
            n191 = Cluster To Array(cluster=w536) -> (array=w533:refnum<vi>[])
            n192 = Build Array (concatenate)(w544, w543) -> (w531:refnum<vi>[])
            n193 = Build Array (concatenate)(w535, w534, w533, w530) -> (w532:refnum<vi>[])
            n194 = call <vilib>:"Clear Errors.vi"("error in (no error)"=w527) -> ("error out"=w529:errorcluster)  [unwired: 5 in, 1 out]
            n195 = call "Enable or Disable UI.vi"("Action"=T14."Enabled", "Error In"=w529, "Control Refs"=w532) -> ("Error Out"=w539:errorcluster)  [unwired: 8 in]
            n196 = call "Enable or Disable UI.vi"("Action"=T14."Disabled", "Error In"=w539, "Control Refs"=w531) -> ("Error Out"=w528:errorcluster)  [unwired: 8 in]
            n197 = Merge Errors(w528, w527) -> (w575:errorcluster)
          }
          frame "Transfer Matrices" {
            # "We dont want this error \nto prevent UI from being \nenabled so we ignore the \nerror."
            # "Transfer the eHS matrices to the deployment target."
            n198 = Unbundle By Name(w595) -> ("Session Init Refs"=w630:T7, "Info Extraction Refs"=w629:T6, "Session R\\C Refs"=w626:T9, "Transfer Netlist(s)"=w624:refnum<vi>, "Matrix Gen Refs"=w621:T8, "General Refs"=w622:T5)
            n199 = Cluster To Array(cluster=w626) -> (array=w625:refnum<vi>[])
            n200 = Cluster To Array(cluster=w630) -> (array=w628:refnum<vi>[])
            n201 = Cluster To Array(cluster=w629) -> (array=w627:refnum<vi>[])
            n202 = Cluster To Array(cluster=w621) -> (array=w620:refnum<vi>[])
            n203 = Cluster To Array(cluster=w622) -> (array=w623:refnum<vi>[])
            n204 = Build Array (concatenate)(w623) -> (w615:refnum<vi>[])
            n205 = Build Array (concatenate)(w628, w627, w625, w624, w620) -> (w614:refnum<vi>[])
            n206 = call "Enable or Disable UI.vi"("Action"=T14."Enabled", "Error In"=w617, "Control Refs"=w615) -> ("Error Out"=w618:errorcluster)  [unwired: 8 in]
            n207 = call "Enable or Disable UI.vi"("Action"=T14."Disabled", "Error In"=w618, "Control Refs"=w614) -> ("Error Out"=w613:errorcluster)  [unwired: 8 in]
            n208 = call <vilib>:"eHS Load Matrices to Target.vi"("Error In"=w613, "eHS Matrix Generation Session Ref In"=w612) -> ("Error Out"=w590:errorcluster, "eHS Matrix Generation Session Ref Out"=w611:refnum<data-value>)  [unwired: 8 in]
            n209 = Unbundle By Name(w595) -> ("Session Init Refs"=w606:T7, "Info Extraction Refs"=w605:T6, "Matrix Gen Refs"=w601:T8, "General Refs"=w602:T5, "Session R\\C Refs"=w600:T9, "Transfer Netlist(s)"=w596:refnum<vi>)
            n210 = Cluster To Array(cluster=w606) -> (array=w604:refnum<vi>[])
            n211 = Cluster To Array(cluster=w605) -> (array=w603:refnum<vi>[])
            n212 = Cluster To Array(cluster=w601) -> (array=w599:refnum<vi>[])
            n213 = Cluster To Array(cluster=w602) -> (array=w598:refnum<vi>[])
            n214 = Cluster To Array(cluster=w600) -> (array=w597:refnum<vi>[])
            n215 = Build Array (concatenate)(w604, w603) -> (w593:refnum<vi>[])
            n216 = Build Array (concatenate)(w599, w598, w597, w596) -> (w594:refnum<vi>[])
            n217 = call <vilib>:"Clear Errors.vi"("error in (no error)"=w590) -> ("error out"=w591:errorcluster)  [unwired: 5 in, 1 out]
            n218 = call "Enable or Disable UI.vi"("Action"=T14."Enabled", "Error In"=w591, "Control Refs"=w594) -> ("Error Out"=w608:errorcluster)  [unwired: 8 in]
            n219 = call "Enable or Disable UI.vi"("Action"=T14."Disabled", "Error In"=w608, "Control Refs"=w593) -> ("Error Out"=w592:errorcluster)  [unwired: 8 in]
            n220 = Merge Errors(w592, w590) -> (w587:errorcluster)
            n221 = call-poly "Enqueue Message.vi"("Error In"=w587, "Message Data"="Transfer complete." ("Message"), "Message"="Update Display", "Message Queue"=w585) -> ("Error Out"=w586:errorcluster)  [unwired: 6 in, 1 out]
          }
          frame "Reset Session" {
            w636 = T3[] [] items=["Core 1", "Core 2", "Core 3", "Core 4", "Core 5", "Core 6", "Core 7", "Core 8", "Core 9", "Core 10"]
            # "Reset eHS Matrix Generation Session"
            n222 = Unbundle By Name(w642) -> ("eHS Listbox"=w633:refnum<vi>, "Session Init Refs"=w648:T7, "Matrix Gen Refs"=w657:T8, "Info Extraction Refs.Extract Model(s) Info"=w637:refnum<vi>, "Transfer Netlist(s)"=w632:refnum<vi>, "Info Extraction Refs"=w650:T6, "Session R\\C Refs"=w644:T9)
            n223 = call <vilib>:"eHS Clear Matrix Generation Session.vi"("Error In"=w640, "eHS Matrix Generation Session In"=w641) -> ("Error Out"=w639:errorcluster, "eHS Matrix Generation Session Ref Out"=w638:refnum<data-value>)  [unwired: 8 in]
            n224 = Cluster To Array(cluster=w648) -> (array=w647:refnum<vi>[])
            n225 = Cluster To Array(cluster=w657) -> (array=w656:refnum<vi>[])
            n226 = Cluster To Array(cluster=w650) -> (array=w649:refnum<vi>[])
            n227 = Cluster To Array(cluster=w644) -> (array=w643:refnum<vi>[])
            n228 = Build Array (concatenate)(w647, w656, w637, w632) -> (w653:refnum<vi>[])
            n229 = Build Array (concatenate)(w649, w643) -> (w655:refnum<vi>[])
            n230 = call "Enable or Disable UI.vi"("Action"=T14."Enabled", "Error In"=w639, "Control Refs"=w655) -> ("Error Out"=w651:errorcluster)  [unwired: 8 in]
            n231 = call "Enable or Disable UI.vi"("Action"=T14."Disabled", "Error In"=w651, "Control Refs"=w653) -> ("Error Out"=w635:errorcluster)  [unwired: 8 in]
            n232 = call "Create ListBox.vi"("Error In"=w635, "Multicolumn Listbox Ref In"=w633) -> ("Error Out"=w634:errorcluster)  [unwired: 8 in, 1 out]
            n233 = call-poly "Enqueue Message.vi"("Error In"=w634, "Message Data"="Session successfully reset. All models in this session have been unloaded. " ("Message"), "Message"="Update Display", "Message Queue"=w645) -> ("Error Out"=w646:errorcluster)  [unwired: 6 in, 1 out]
            n234 = Merge Errors(w646) -> (w661:errorcluster)
          }
          frame "Close Session" {
            w666 = T3[] [] items=["Core 1", "Core 2", "Core 3", "Core 4", "Core 5", "Core 6", "Core 7", "Core 8", "Core 9", "Core 10"]
            # "We dont care if \nthe ref is invalid"
            # "Close eHS Matrix Generation Session"
            n235 = Unbundle By Name(w677) -> ("eHS Listbox"=w663:refnum<vi>, "Session Init Refs"=w682:T7, "General Refs"=w691:T5, "Info Extraction Refs"=w684:T6, "Matrix Gen Refs"=w674:T8, "Session R\\C Refs"=w673:T9, "Transfer Netlist(s)"=w671:refnum<vi>)
            n236 = Cluster To Array(cluster=w682) -> (array=w681:refnum<vi>[])
            n237 = Cluster To Array(cluster=w691) -> (array=w690:refnum<vi>[])
            n238 = Cluster To Array(cluster=w684) -> (array=w683:refnum<vi>[])
            n239 = Cluster To Array(cluster=w674) -> (array=w678:refnum<vi>[])
            n240 = Cluster To Array(cluster=w673) -> (array=w672:refnum<vi>[])
            n241 = call <vilib>:"eHS Close Matrix Generation Session.vi"("Error In"=w675, "eHS Matrix Generation Session Ref In"=w676) -> ("Error Out"=w669:errorcluster)  [unwired: 9 in]
            n242 = Build Array (concatenate)(w681, w690) -> (w687:refnum<vi>[])
            n243 = Build Array (concatenate)(w683, w678, w672, w671) -> (w689:refnum<vi>[])
            n244 = call <vilib>:"Clear Errors.vi"("error in (no error)"=w669, "specific error code to clear (0: all)"=1556) -> ("error out"=w668:errorcluster)  [unwired: 4 in, 1 out]
            n245 = call "Enable or Disable UI.vi"("Action"=T14."Disabled", "Error In"=w668, "Control Refs"=w689) -> ("Error Out"=w685:errorcluster)  [unwired: 8 in]
            n246 = call "Enable or Disable UI.vi"("Action"=T14."Enabled", "Error In"=w685, "Control Refs"=w687) -> ("Error Out"=w665:errorcluster)  [unwired: 8 in]
            n247 = call "Create ListBox.vi"("Error In"=w665, "Multicolumn Listbox Ref In"=w663) -> ("Error Out"=w664:errorcluster)  [unwired: 8 in, 1 out]
            n248 = call-poly "Enqueue Message.vi"("Priority Message? (F)"=FALSE, "Error In"=w664, "Message Data"="Session successfully closed." ("Message"), "Message"="Update Display", "Message Queue"=w679) -> ("Error Out"=w680:errorcluster)  [unwired: 5 in, 1 out]
            n249 = Merge Errors(w680) -> (w695:errorcluster)
          }
          frame "Get Report" {
            # "Display the eHS matrix build log to the user"
            n250 = call <vilib>:"Application Directory.vi"() -> ("Application Directory"=w705:path)
            n251 = Build Path(base path=w705, name or relative path="eHS Matrix Build Log\\eHS Matrix Build Log.txt ") -> (appended path=w703:path)
            n252 = Read from Text File(file (use dialog)=w703, error in=w702) -> (text=→"eHS Generation Reports":string, error out=w698:errorcluster)  [unwired: 2 in, 2 out]
            n253 = case shown="No Error" w698 {
              selector: w698 -> [w707 _]
              tunnel: [w711 w712] -> w700
              tunnel: w699 -> [w710 _]
              frame No Error {
                n254 = call-poly "Enqueue Message.vi"("Error In"=w707, "Message Data"="Log Retreived" ("Message"), "Message"="Update Display", "Message Queue"=w710) -> ("Error Out"=w711:errorcluster)  [unwired: 6 in, 1 out]
              }
              frame Error {
                n255 = xnode "Error Ring"() -> ("error out"=w712:errorcluster)
              }
            }
          }
          frame "Display Help" {
            # "WE will need to change this. Not very elegant locks entire UI."
            n256 = call "Help.vi"("Error In"=w719) -> ("Error Out"=w718:errorcluster)  [unwired: 10 in]
            n257 = Merge Errors(w718) -> (w723:errorcluster)
          }
          frame "Confirm Quit" {
            # "#CodeNeeded - If you want to provide an \"Are you sure\" dialog (or some other notification) before the application exits, place that code here. This message is typically sent from a Panel Close? event."
            # "Confirm Quit - Message that can confirm whether or not the user wants to exit the application."
            n258 = call-poly "Enqueue Message.vi"("Error In"=w731, "Message Data"="Exiting Program..." ("Message"), "Message"="Update Display", "Message Queue"=w732) -> ("Error Out"=w727:errorcluster, "dup Message Queue"=w729:refnum<queue>)  [unwired: 6 in]
            n259 = call-poly "Enqueue Message.vi"("Error In"=w727, "Message"="Close Session", "Message Queue"=w729) -> ("Error Out"=w726:errorcluster, "dup Message Queue"=w728:refnum<queue>)  [unwired: 7 in]
            n260 = call-poly "Enqueue Message.vi"("Error In"=w726, "Message"="Exit", "Message Queue"=w728) -> ("Error Out"=w738:errorcluster)  [unwired: 7 in, 1 out]
            n261 = Merge Errors(w738) -> (w739:errorcluster)
          }
          frame "Exit" {
            w741 = T3[] [] items=["Core 1", "Core 2", "Core 3", "Core 4", "Core 5", "Core 6", "Core 7", "Core 8", "Core 9", "Core 10"]
            # "Stop the VI"
            # "Release the message queue reference"
            # "#CodeNeeded - Add any required cleanup code here. Note that if 'Exit' was called as a result of an error, an error dialog will be displayed. Add any custom error handling for an 'Exit' condition here as well."
            # "Exit - Exit the application."
            n262 = Variant To Data(type=errorcluster {"status"=FALSE, "code"=0, "source"=""} ("error constant"), Variant=w745) -> (data=w746:errorcluster)  [unwired: 1 in, 1 out]
            n263 = call <vilib>:"Simple Error Handler.vi"("error in (no error)"=w746) -> ()  [unwired: 4 in, 5 out]
            n264 = call "Fire User Event - Stop.vi"("User Event - Stop"=w750) -> ("Error out"=w749:errorcluster)  [unwired: 10 in]
            n265 = Release Queue(queue=w753, error in (no error)=w748) -> (error out=w743:errorcluster)  [unwired: 1 in, 2 out]
            n266 = Merge Errors(w749, w743) -> (w751:errorcluster)
          }
          frame "Error" {
            # "#CodeRecommended - If you ever change the name of this \"Error\" message, you'll need to update the name in the Check Loop Error.vi as well."
            # "#CodeRecommended - Consider creating a system for logging errors in some way. These errors are for notification purposes only. Handling of specific errors should be performed in the message frames that generated the error."
            # "Error - Display an error dialog. This message is sent by the \"Error Handler\" VIs at the end of other loops in this application."
            n267 = Variant To Data(error in=w763, type=errorcluster {"status"=FALSE, "code"=0, "source"=""} ("error constant"), Variant=w761) -> (data=w759:errorcluster, error out=w758:errorcluster)
            n268 = call <vilib>:"Simple Error Handler.vi"("error in (no error)"=w759) -> ()  [unwired: 4 in, 5 out]
            n269 = Merge Errors(w758) -> (w757:errorcluster)
          }
          frame "---Copy This Frame---" {
            # "Duplicate this frame when creating new messages.  Change this comment in the duplicated frame to describe this message."
            n270 = Merge Errors(w767) -> (w765:errorcluster)
          }
          frame Default {
            # "'Default' case only runs if there is a message that isn't defined in any of the other cases.  Output a programming error."
            n271 = xnode "Error Ring"("parameter 0"=w771) -> ("error out"=w772:errorcluster)
          }
        }
        n272 = call "Error Handler - Message Handling Loop.vi"("error in (no error)"=w132, "Message Queue"=w134) -> ("dup error in"=w133:errorcluster)  [unwired: 8 in, 1 out]
      }
      n273 = while {
        tunnel: w15 -> [w25]
        shift-right: [w23] -> w11
        shift-left: w9 -> [w24]
        tunnel: [w19] -> w10
        stop <- w21 stop-if-true
        # "Event Handling Loop - User Inputs"
        n274 = event shown="[3] \"Extract Model(s) Info\": Value Change" {
          selector: w24 -> [_ _ _ _ _ _ _ _ _ _ _ _ _ _ _]
          dyn-events: [_ _ _ _ _ _ _ _ _ _ _ _ _ _ _] -> w23
          timeout: _ -> [_ _ _ _ _ _ _ _ _ _ _ _ _ _ _]
          tunnel: [FALSE ("Discard?") FALSE ("Discard?") FALSE ("Discard?") FALSE ("Discard?") FALSE ("Discard?") FALSE ("Discard?") FALSE ("Discard?") _ FALSE ("Discard?") FALSE ("Discard?") FALSE ("Discard?") FALSE ("Discard?") FALSE ("Discard?") FALSE ("Discard?") TRUE ("Discard?")] -> w21
          tunnel: w25 -> [w35 w50 w55 w64 w73 w78 w82 w88 w96 w101 w105 w113 w116 w120 w127]
          tunnel: [w36 w47 w56 w66 w70 w75 w85 w90 w93 w98 w103 w112 _ w123 _] -> w22
          tunnel: [w37 w49 w57 w68 w72 w77 w87 w89 w95 w100 w104 w111 w116 w125 w127] -> w20
          event "Create Session": Value Change {
            n275 = event-data() -> ()  [unwired: 1 in, 1 out]
            n276 = call-poly "Enqueue Message.vi"("Message Data"="Creating session and verifying if deployment target is online..." ("Message"), "Message"="Update Display", "Message Queue"=w35) -> ("Error Out"=w33:errorcluster, "dup Message Queue"=w34:refnum<queue>)  [unwired: 7 in]
            n277 = Bundle By Name(cluster=T10 {"Deployment Target"="", "Username"="", "Password"=""} ("eHS Target Information"), "Deployment Target"="Deployment Target", "Username"="Target Username", "Password"="Target Password") -> (w29:T10)
            n278 = call-poly "Enqueue Message.vi"("Error In"=w33, "Message Data"=w29, "Message"="Create Session", "Message Queue"=w34) -> ("Error Out"=w36:errorcluster, "dup Message Queue"=w37:refnum<queue>)  [unwired: 6 in]
          }
          event "Add Model": Value Change {
            n279 = event-data() -> ()  [unwired: 1 in, 1 out]
            n280 = Bundle By Name(cluster=T11 {"eHS Core Settings"={"eHS Form Factor"=enum."eHSx16", "eHS Core Index"=enum."Core 1"}, "eHS Model Information"={"Model File Path"=path "", "Model Name"="", "Model File Extension"="", "Senarios?"=FALSE}} ("Info to Add Model"), "eHS Core Settings.eHS Core Index"="eHS Core Index", "eHS Core Settings.eHS Form Factor"="eHS Form Factor", "eHS Model Information.Model File Path"="Model Location On Disk", "eHS Model Information.Senarios?"="Support Scenarios?") -> (w41:T11)
            n281 = call-poly "Enqueue Message.vi"("Message Data"=w41, "Message"="Add Model", "Message Queue"=w50) -> ("Error Out"=w47:errorcluster, "dup Message Queue"=w49:refnum<queue>)  [unwired: 7 in]
          }
          event "Add Model(s)-File": Value Change {
            n282 = event-data() -> ()  [unwired: 1 in, 1 out]
            n283 = call-poly "Enqueue Message.vi"("Message Data"="Adding models from file..." ("Message"), "Message"="Update Display", "Message Queue"=w55) -> ("Error Out"=w53:errorcluster, "dup Message Queue"=w54:refnum<queue>)  [unwired: 7 in]
            n284 = call-poly "Enqueue Message.vi"("Error In"=w53, "Message"="Add Model(s) - File", "Message Queue"=w54) -> ("Error Out"=w56:errorcluster, "dup Message Queue"=w57:refnum<queue>)  [unwired: 7 in]
          }
          event "Extract Model(s) Info": Value Change {
            n285 = event-data() -> ()  [unwired: 1 in, 1 out]
            n286 = call-poly "Enqueue Message.vi"("Message Data"="Determining number of models for extraction...  " ("Message"), "Message"="Update Display", "Message Queue"=w64) -> ("Error Out"=w62:errorcluster, "dup Message Queue"=w63:refnum<queue>)  [unwired: 7 in]
            n287 = call-poly "Enqueue Message.vi"("Error In"=w62, "Message"="Init Extract Model(s)", "Message Queue"=w63) -> ("Error Out"=w66:errorcluster, "dup Message Queue"=w68:refnum<queue>)  [unwired: 7 in]
          }
          event "Update Settings": Value Change {
            n288 = event-data() -> ()  [unwired: 1 in, 1 out]
            n289 = call-poly "Enqueue Message.vi"("Message"="Update Settings", "Message Queue"=w73) -> ("Error Out"=w70:errorcluster, "dup Message Queue"=w72:refnum<queue>)  [unwired: 8 in]
          }
          event "Generate Matrix(s)": Value Change {
            n290 = event-data() -> ()  [unwired: 1 in, 1 out]
            n291 = call-poly "Enqueue Message.vi"("Message"="Init Generate Matrices", "Message Queue"=w78) -> ("Error Out"=w75:errorcluster, "dup Message Queue"=w77:refnum<queue>)  [unwired: 8 in]
          }
          event "Transfer Matrices": Value Change {
            n292 = event-data() -> ()  [unwired: 1 in, 1 out]
            n293 = call-poly "Enqueue Message.vi"("Message Data"="Tranfering eHS Matrices to the target..." ("Message"), "Message"="Update Display", "Message Queue"=w82) -> ("Error Out"=w80:errorcluster, "dup Message Queue"=w81:refnum<queue>)  [unwired: 7 in]
            n294 = call-poly "Enqueue Message.vi"("Error In"=w80, "Message"="Transfer Matrices", "Message Queue"=w81) -> ("Error Out"=w85:errorcluster, "dup Message Queue"=w87:refnum<queue>)  [unwired: 7 in]
          }
          event "Get Report": Value Change {
            n295 = event-data() -> ()  [unwired: 1 in, 1 out]
            n296 = call-poly "Enqueue Message.vi"("Message"="Get Report", "Message Queue"=w88) -> ("Error Out"=w90:errorcluster, "dup Message Queue"=w89:refnum<queue>)  [unwired: 8 in]
          }
          event "Reset Session": Value Change {
            n297 = event-data() -> ()  [unwired: 1 in, 1 out]
            n298 = call-poly "Enqueue Message.vi"("Message"="Reset Session", "Message Queue"=w96) -> ("Error Out"=w93:errorcluster, "dup Message Queue"=w95:refnum<queue>)  [unwired: 8 in]
          }
          event "Close Session": Value Change {
            n299 = event-data() -> ()  [unwired: 1 in, 1 out]
            n300 = call-poly "Enqueue Message.vi"("Message"="Close Session", "Message Queue"=w101) -> ("Error Out"=w98:errorcluster, "dup Message Queue"=w100:refnum<queue>)  [unwired: 8 in]
          }
          event "Quit Button": Value Change {
            n301 = event-data() -> ()  [unwired: 1 in, 1 out]
            n302 = call-poly "Enqueue Message.vi"("Priority Message? (F)"=TRUE, "Message"="Confirm Quit", "Message Queue"=w105) -> ("Error Out"=w103:errorcluster, "dup Message Queue"=w104:refnum<queue>)  [unwired: 7 in]
          }
          event Panel Close? {
            n303 = event-data() -> ()  [unwired: 1 in, 1 out]
            n304 = call-poly "Enqueue Message.vi"("Priority Message? (F)"=TRUE, "Message"="Confirm Quit", "Message Queue"=w113) -> ("Error Out"=w112:errorcluster, "dup Message Queue"=w111:refnum<queue>)  [unwired: 7 in]
            n305 = event-data("Discard?"=TRUE) -> ()  [unwired: 1 in, 1 out]
          }
          event Application Instance Close {
            # "#CodeRecommended - When a project closes, all VIs within that project are aborted and leave memory. However, any code placed in this event frame is guaranteed to run to completion, so add any cleanup code that absolutely must happen here."
            n306 = event-data() -> ()  [unwired: 1 in, 1 out]
          }
          event "Help Button": Value Change {
            n307 = event-data() -> ()  [unwired: 1 in, 1 out]
            n308 = call-poly "Enqueue Message.vi"("Message Data"="Opening Help..." ("Message"), "Message"="Update Display", "Message Queue"=w120) -> ("Error Out"=w121:errorcluster, "dup Message Queue"=w119:refnum<queue>)  [unwired: 7 in]
            n309 = call-poly "Enqueue Message.vi"("Error In"=w121, "Message"="Display Help", "Message Queue"=w119) -> ("Error Out"=w123:errorcluster, "dup Message Queue"=w125:refnum<queue>)  [unwired: 7 in]
          }
          event User Event {
            # "The Message Handling Loop processed an \"Exit\" message, which fired this event to stop the Event Handling Loop."
            n310 = event-data() -> ()  [unwired: 1 in, 1 out]
          }
        }
        n311 = call "Error Handler - Event Handling Loop.vi"("Error In"=w22, "Message Queue"=w20) -> ("dup Error Out"=w19:errorcluster)  [unwired: 8 in, 1 out]
      }
      n312 = Unregister For Events(event registration refnum=w11, error in=w10) -> (error out=w12:errorcluster)
      n313 = Merge Errors(w12, w16) -> (w13:errorcluster)
      n314 = call "Destroy User Event - Stop.vi"("error in (no error)"=w13, "User Event - Stop"=w8) -> ("error out"=w4:errorcluster)  [unwired: 9 in]
    }
    frame Error {
    }
  }
  "error out" <- w2
